vi "FT10_Log LVM Values.vi"(8 "error in (no error)":errorcluster, 10 "Log Cluster in":T2, 11 "Log Loop Cluster in":T13={"tdms file out"=refnum, "t0"="", "Generator Serial Number in"="T1234567DX"}) -> (0 "error out":errorcluster, 1 "Filename Cluster out":T1, 2 "Log Cluster out":T2, 3 "Log Loop Cluster out":T13={"tdms file out"=refnum, "t0"="", "Generator Serial Number in"="T1234567DX"})   [LabVIEW 2024]
doc: "Saves current and diff voltage to LVM files each time measuremnet is taken."
uses:
  Controls/Control_Log Loop Cluster.ctl
  Controls/Control_Log TDMS Filename.ctl
  Controls/Control_Log t0.ctl
  Controls/Control_Serial Number.ctl
  Controls/Control_Log Cluster.ctl
  Controls/Control_Log Time.ctl
  Controls/Control_Log Waveform Cluster - Current.ctl
  Controls/Control_Log Analysis Cluster - Current.ctl
  Controls/Control_Log Activation Settings Cluster.ctl
  Controls/Control_Log Unitherm Load.ctl
  Controls/Control_Log Port.ctl
  Controls/Control_Log Mode.ctl
  Controls/Control_Log Power Level.ctl
  Controls/Control_Log Waveform Cluster - Diff Voltage.ctl
  Controls/Control_Log Analysis Cluster - Diff Voltage.ctl
  Controls/Control_Log Filename Cluster.ctl
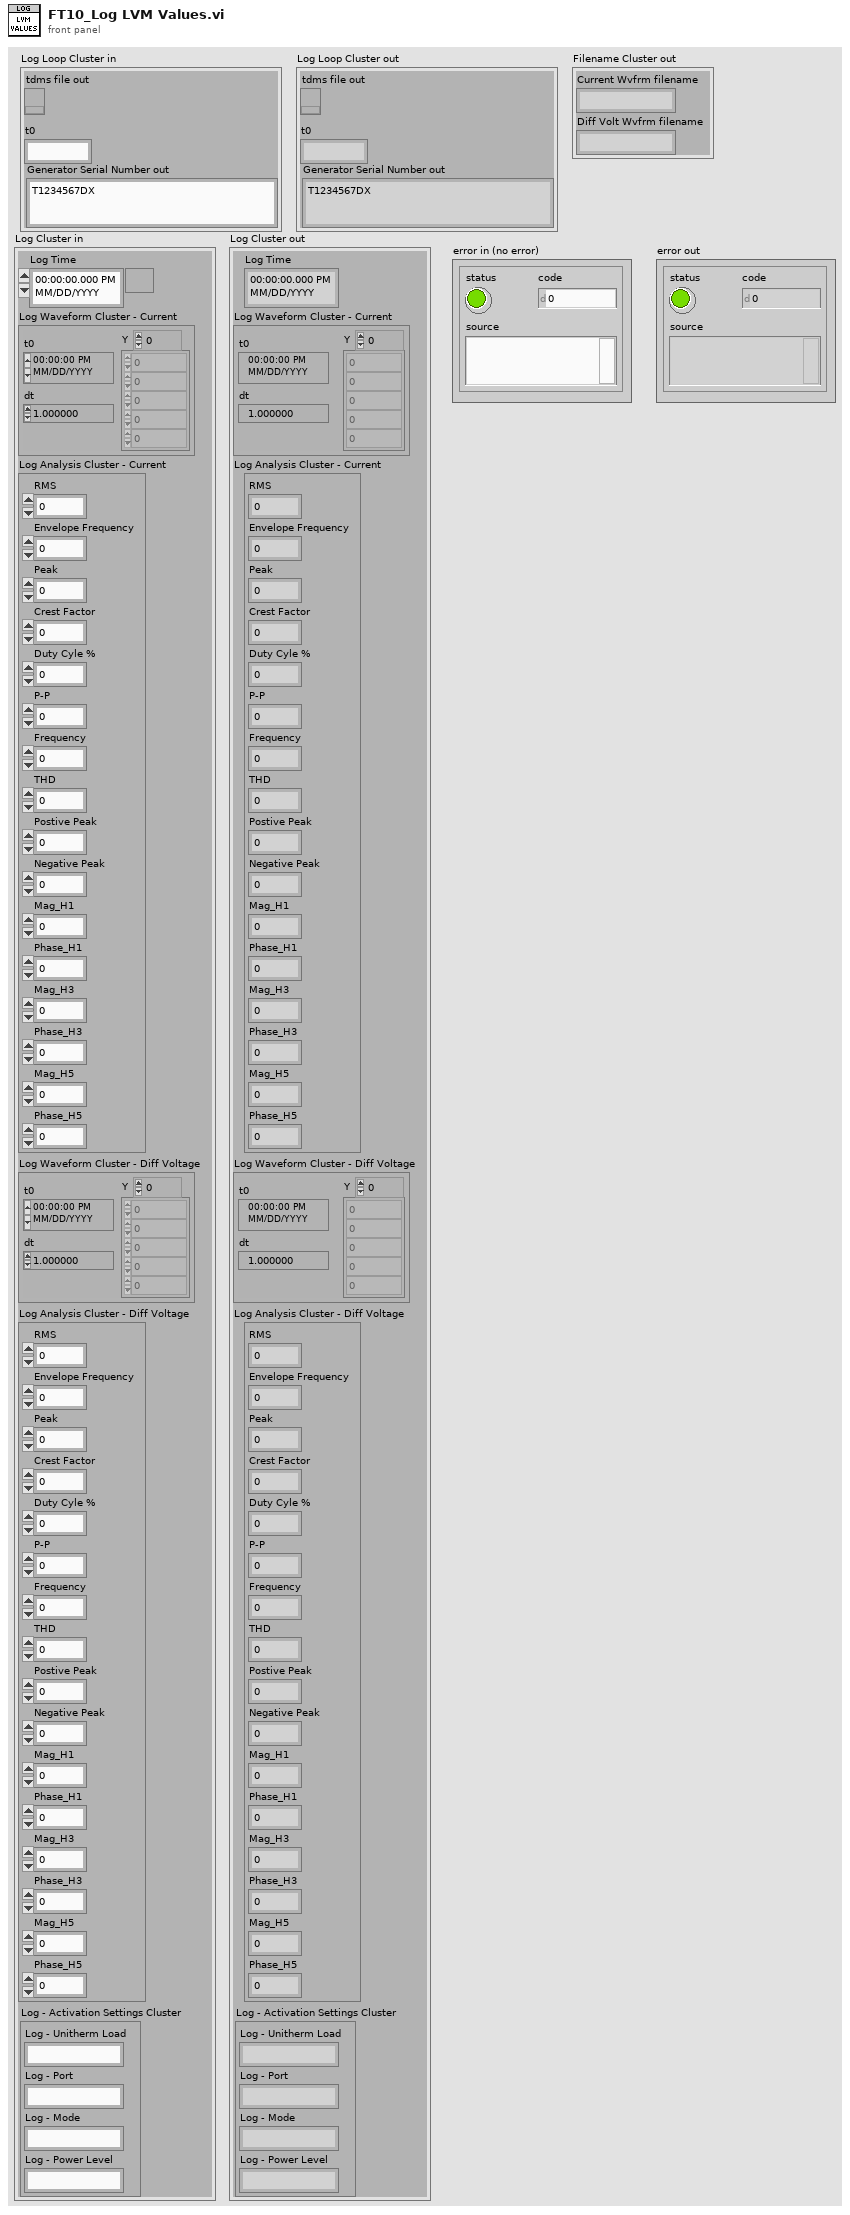
[diagram p1: front panel]
types:
  T1 = typedef "Control_Log Filename Cluster.ctl" = cluster{"Current Wvfrm filename":string, "Diff Volt Wvfrm filename":string}
  T2 = typedef "Control_Log Cluster.ctl" = cluster{"Log Time":T3, "Log Waveform Cluster - Current":T4, "Log Analysis Cluster - Current":T5, "Log - Activation Settings Cluster":T6, "Log Waveform Cluster - Diff Voltage":T11, "Log Analysis Cluster - Diff Voltage":T12}
  T3 = typedef "Control_Log Time.ctl" = timestamp
  T4 = typedef "Control_Log Waveform Cluster - Current.ctl" = waveform(dbl)
  T5 = typedef "Control_Log Analysis Cluster - Current.ctl" = cluster{"RMS":dbl, "Envelope Frequency":dbl, "Peak":dbl, "Crest Factor":dbl, "Duty Cyle %":dbl, "P-P":dbl, "Frequency":dbl, "THD":dbl, "Postive Peak":dbl, "Negative Peak":dbl, "Mag_H1":dbl, "Phase_H1":dbl, "Mag_H3":dbl, "Phase_H3":dbl, "Mag_H5":dbl, "Phase_H5":dbl}
  T6 = typedef "Control_Log Activation Settings Cluster.ctl" = cluster{"Log - Unitherm Load":T7, "Log - Port":T8, "Log - Mode":T9, "Log - Power Level":T10}
  T7 = typedef "Control_Log Unitherm Load.ctl" = string
  T8 = typedef "Control_Log Port.ctl" = string
  T9 = typedef "Control_Log Mode.ctl" = string
  T10 = typedef "Control_Log Power Level.ctl" = string
  T11 = typedef "Control_Log Waveform Cluster - Diff Voltage.ctl" = waveform(dbl)
  T12 = typedef "Control_Log Analysis Cluster - Diff Voltage.ctl" = cluster{"RMS":dbl, "Envelope Frequency":dbl, "Peak":dbl, "Crest Factor":dbl, "Duty Cyle %":dbl, "P-P":dbl, "Frequency":dbl, "THD":dbl, "Postive Peak":dbl, "Negative Peak":dbl, "Mag_H1":dbl, "Phase_H1":dbl, "Mag_H3":dbl, "Phase_H3":dbl, "Mag_H5":dbl, "Phase_H5":dbl}
  T13 = typedef "Control_Log Loop Cluster.ctl" = cluster{"tdms file out":T14, "t0":T15, "Generator Serial Number in":T16}
  T14 = typedef "Control_Log TDMS Filename.ctl" = refnum<k34>
  T15 = typedef "Control_Log t0.ctl" = string
  T16 = typedef "Control_Serial Number.ctl" = string
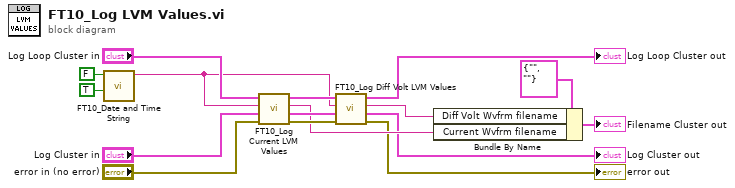
[diagram p0: block diagram]
diagram:
  n1 = call "FT10_Date and Time String.vi"("Include msec"=TRUE, "to UTC"=FALSE) -> ("Date & Time string"=w6:string)  [unwired: 9 in]
  n2 = call "FT10_Log Current LVM Values.vi"("error in (no error)"="error in (no error)", "Log Cluster in"="Log Cluster in", "Date & Time string"=w6, "Log Loop Cluster in"="Log Loop Cluster in") -> ("error out"=w8:errorcluster, "Log Cluster out"=w9:T2, "Current Wvfrm filename"=w5:string, "Log Loop Cluster out"=w10:T13)  [unwired: 4 in]
  n3 = call "FT10_Log Diff Volt LVM Values.vi"("error in (no error)"=w8, "Log Cluster in"=w9, "Date & Time string"=w6, "Log Loop Cluster in"=w10) -> ("error out"=→"error out":errorcluster, "Log Cluster out"=→"Log Cluster out":T2, "Diff Volt Wvfrm filename"=w4:string, "Log Loop Cluster out"=→"Log Loop Cluster out":T13)  [unwired: 4 in]
  n4 = Bundle By Name(cluster=T1 {"Current Wvfrm filename"="", "Diff Volt Wvfrm filename"=""}, "Diff Volt Wvfrm filename"=w4, "Current Wvfrm filename"=w5) -> (→"Filename Cluster out":T1)
